vi "GenCirc (SubVI).vi"() -> (2 "Cluster":cluster{dbl[], dbl[]})   [LabVIEW 2019]
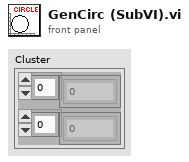
[diagram p1: front panel]
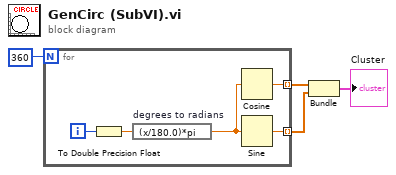
[diagram p0: block diagram]
diagram:
  n1 = for {
    N: 360 -> [_]
    tunnel: [w8] -> w2 mode=indexing
    tunnel: [w7] -> w3 mode=indexing
    i -> [w6]
    n2 = To Double Precision Float(number=w6) -> (double precision float=w5:dbl)
    n3 = expression code="(x/180.0)*pi" "degrees to radians"(w5) -> (w9:dbl)
    n4 = Cosine(x=w9) -> (cos(x)=w8:dbl)
    n5 = Sine(x=w9) -> (sin(x)=w7:dbl)
  }
  n6 = Bundle(w2, w3) -> (→"Cluster":cluster{dbl[], dbl[]})  [unwired: 1 in]
